vi "Read Output.vi"(8 "error in":errorcluster, 10 "byte count":i32=1000, 11 "pipe in":T1) -> (0 "error out":errorcluster, 2 "read buffer":string, 3 "pipe out":T1, 5 "bytes remaining":i32)   [LabVIEW 2013, in "GOLPI library.lvlib"]
uses:
  GOLPI library.lvlib
  LV Process.lvlibp/Pipe Handle.ctl
  LV Process.lvlibp
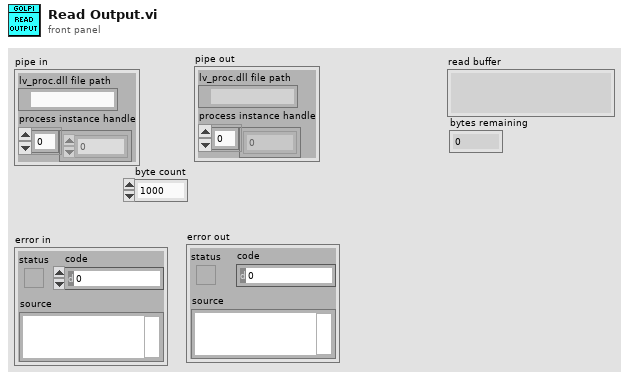
[diagram p1: front panel]
types:
  T1 = typedef "LV Process.lvlibp/Pipe Handle.ctl" = cluster{"lv_proc.dll file path":path, "process instance handle":u32[]}
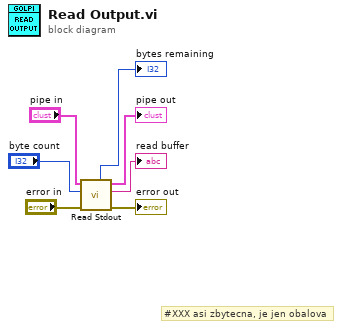
[diagram p0: block diagram]
diagram:
  # "#XXX asi zbytecna, je jen obalova"
  n1 = call "Read Stdout.vi"("error in"="error in", "byte count"="byte count", "pipe in"="pipe in") -> ("error out"=→"error out":errorcluster, "read buffer"=→"read buffer":string, "pipe out"=→"pipe out":T1, "bytes remaining"=→"bytes remaining":i32)  [unwired: 3 in, 2 out]
